vi "Main.vi"(0 "Operation":string(combo), 1 "Delete":bool, 5 "Add":bool, 7 "Load":bool, 9 "Save":bool, 11 "Error In":errorcluster, 12 "Tree":string(tree)) -> (15 "Error Out":errorcluster)   [LabVIEW 2021, in "Calculator.lvlib"]
doc: "This VI acts as a calculator , which has four child classes with the overriding methods and seperate UI VIs for each class which is opened in subpanel when the particular instance is selected. Also the class data is stored in XML file and it can be loaded when required."
uses:
  Calculator.lvlib
  Controls/Queue Operations.ctl
  Classes/NumericOperation/NumericOperation.lvclass
  Controls/Data Cluster.ctl
  Controls/Class Data.ctl
  Controls/User Event Operations.ctl
  <vilib>/Utility/xml.llb/Write to XML File(string).vi
  <vilib>/Utility/xml.llb/Read From XML File(array).vi
panel:
  in  "Help Button":bool
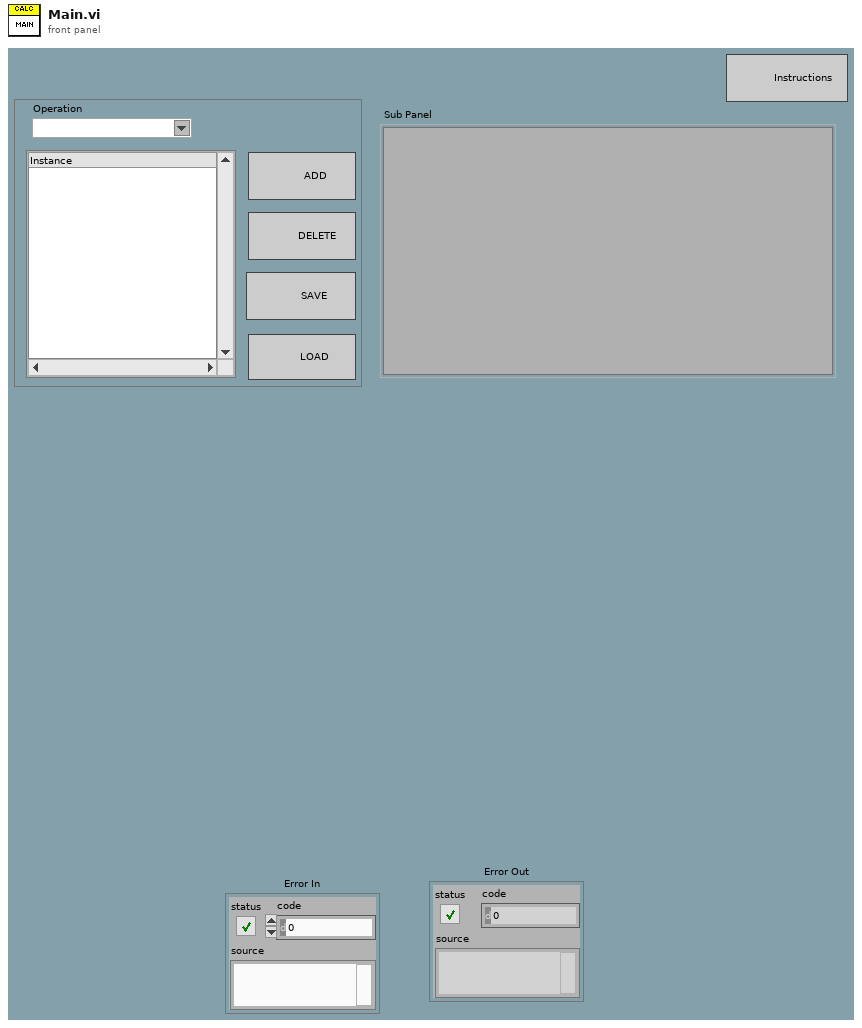
[diagram p1: front panel]
types:
  T1 = typedef "Calculator.lvlib/User Event Operations.ctl" = enum16{"Obtain", "Generate", "Release"}
  T2 = typedef "Calculator.lvlib/Queue Operations.ctl" = enum16{"Create", "Enqueue", "EnqueueN", "Enqueue at top", "Dequeue", "Flush", "Release"}
  T3 = typedef "Calculator.lvlib/Data Cluster.ctl" = cluster{"A":dbl, "B":dbl, "C":dbl, "NumericOperation.lvclass":refnum<class "NumericOperation.lvclass">, "generic class reference":refnum<class "NumericOperation.lvclass">, "Operation":string, "Active Tag":string, "Path":path, "VI Refnum":refnum<vi>, "Class Data":refnum<class "NumericOperation.lvclass">, "DataArray":T4[], "FilePath":path, "Class Name":string, "Data Value Reference Out":refnum<data-value>}
  T4 = typedef "Calculator.lvlib/Class Data.ctl" = cluster{"Class Data":refnum<class "NumericOperation.lvclass">, "String":string}
  T5 = typedef "LVPoint32TypeDef.ctl" = cluster{"Horizontal":i32, "Vertical":i32}
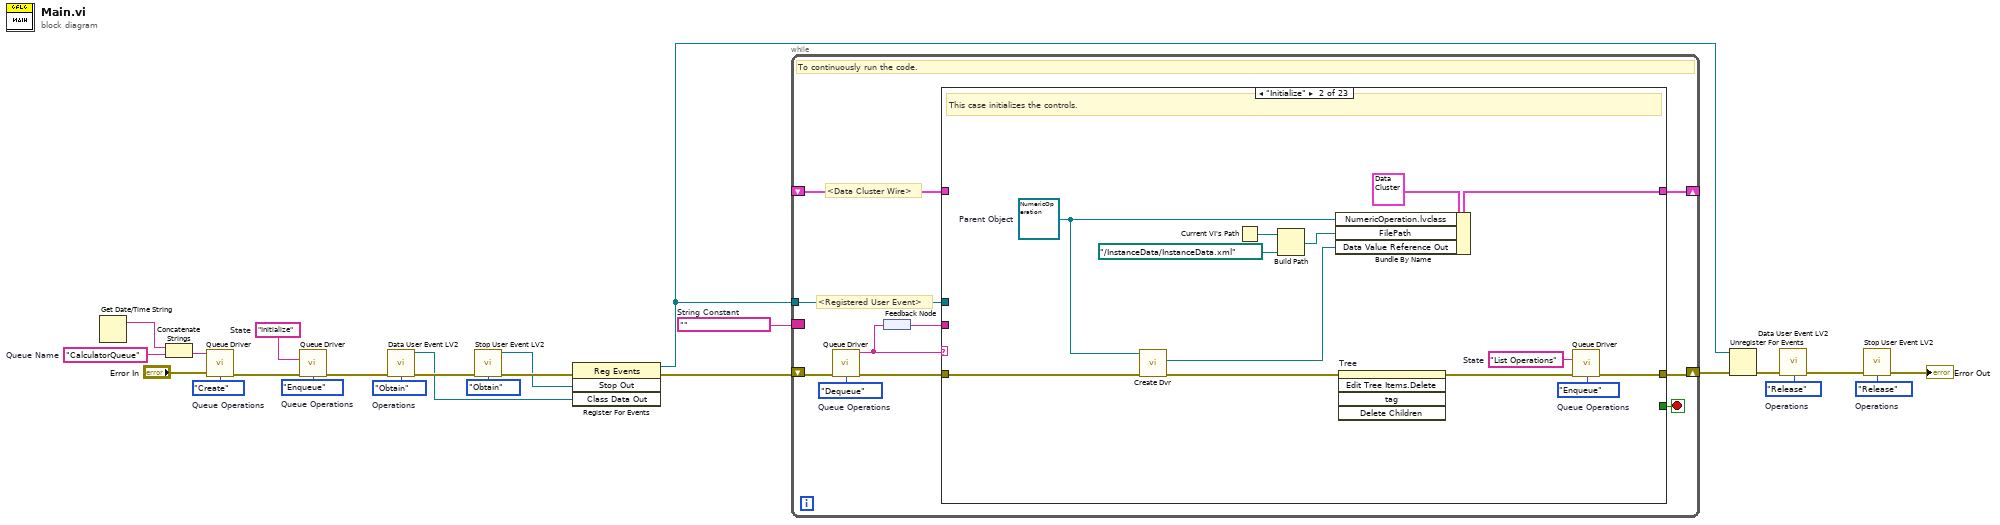
[diagram p0: block diagram]
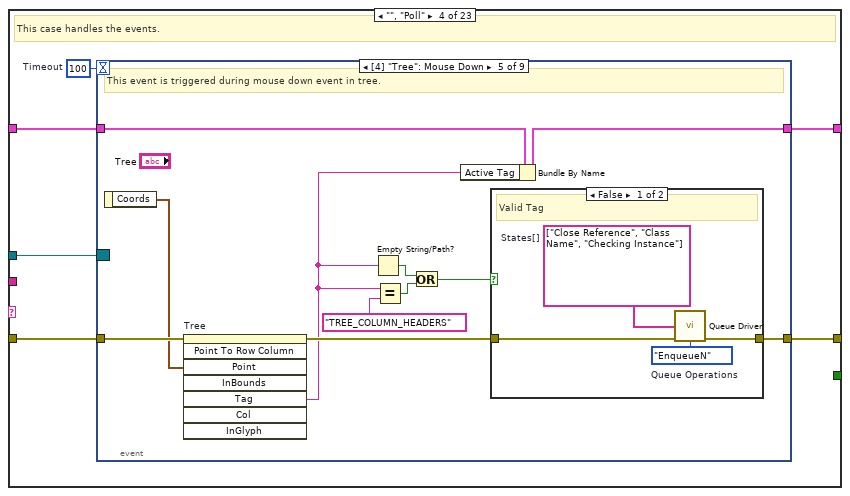
[diagram p4: hidden frame]
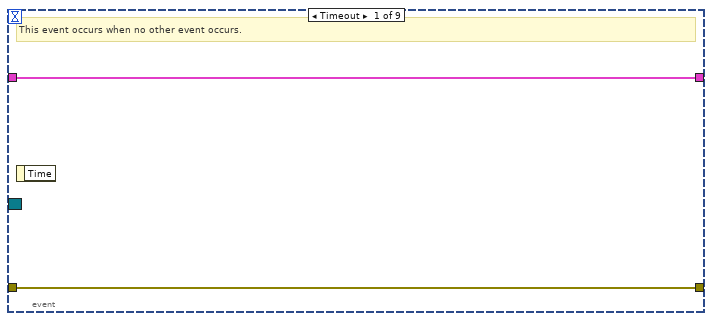
[diagram p5: hidden frame]
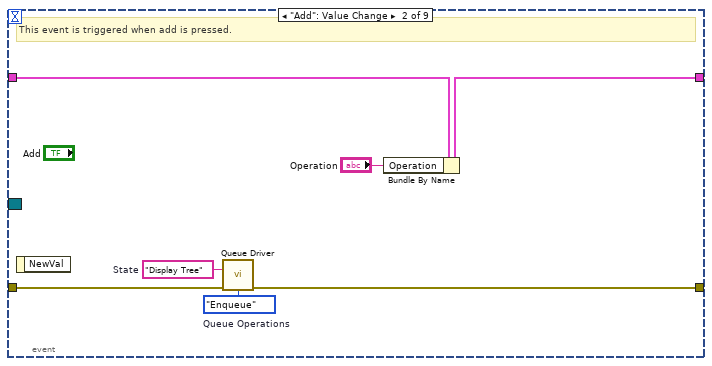
[diagram p6: hidden frame]
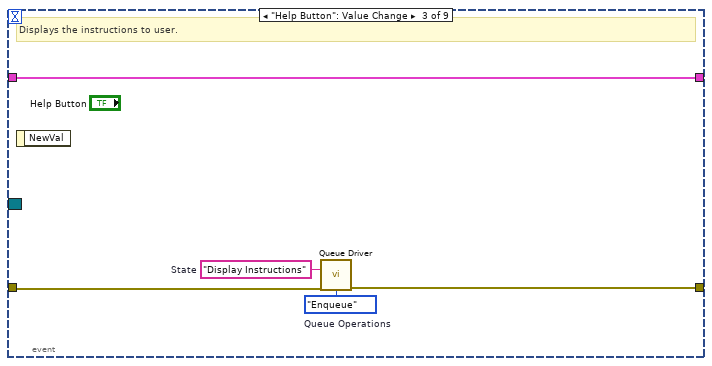
[diagram p7: hidden frame]
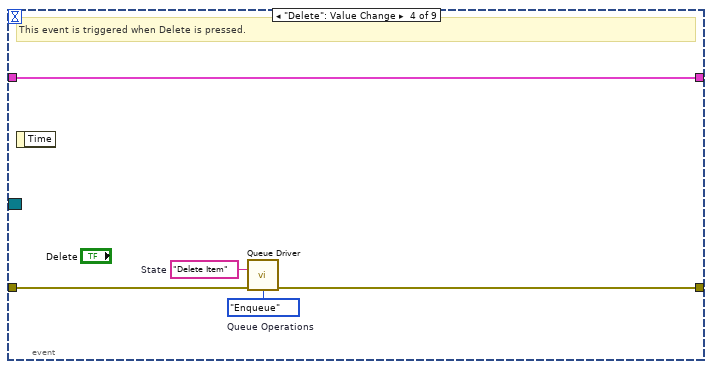
[diagram p8: hidden frame]
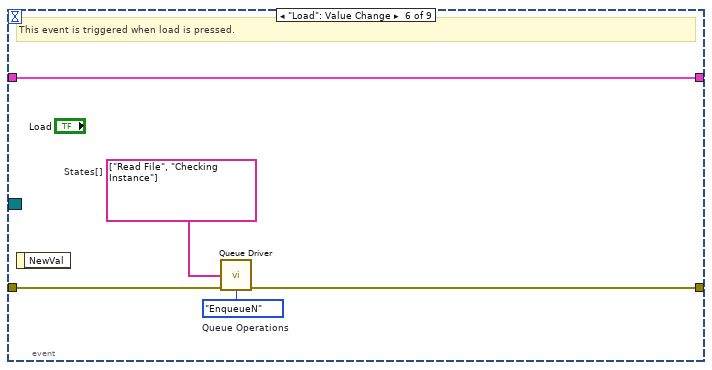
[diagram p10: hidden frame]
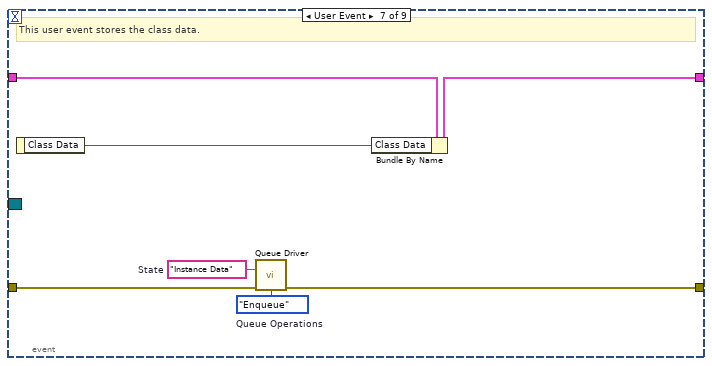
[diagram p11: hidden frame]
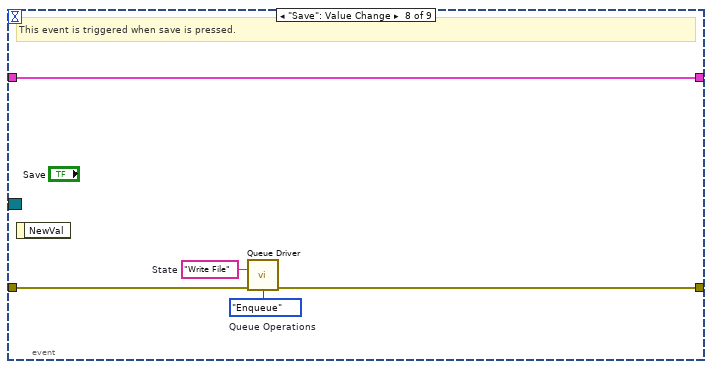
[diagram p12: hidden frame]
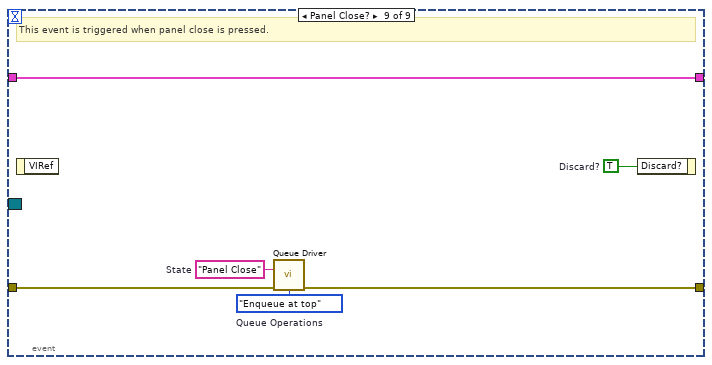
[diagram p13: hidden frame]
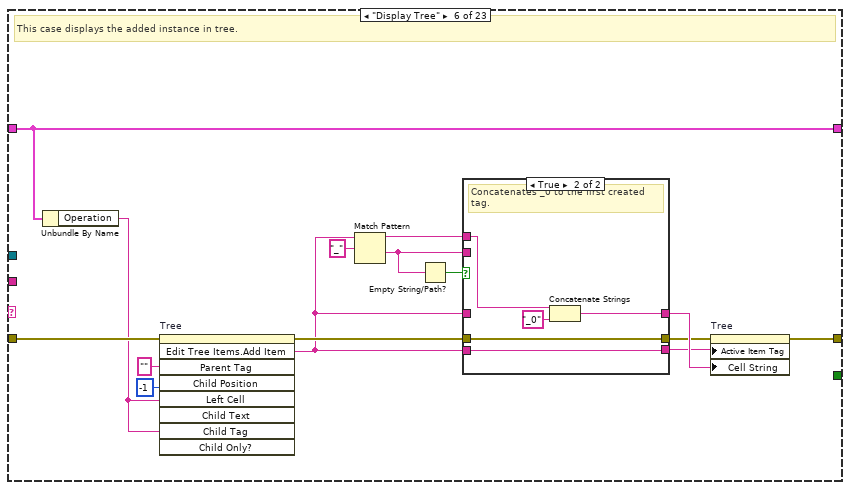
[diagram p15: hidden frame]
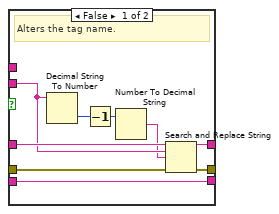
[diagram p16: hidden frame]
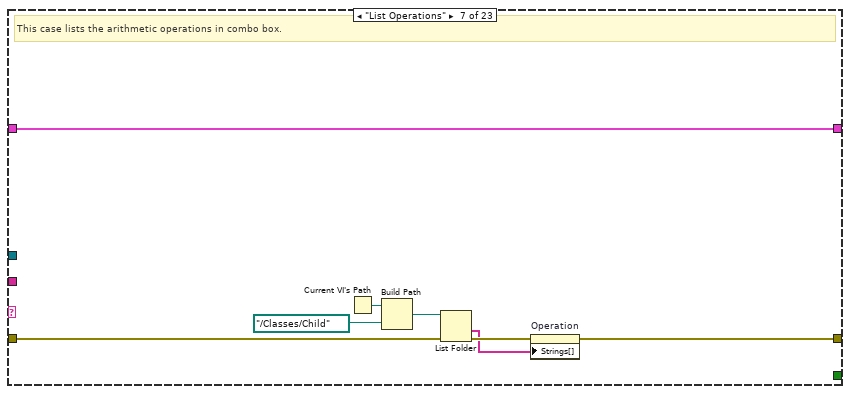
[diagram p17: hidden frame]
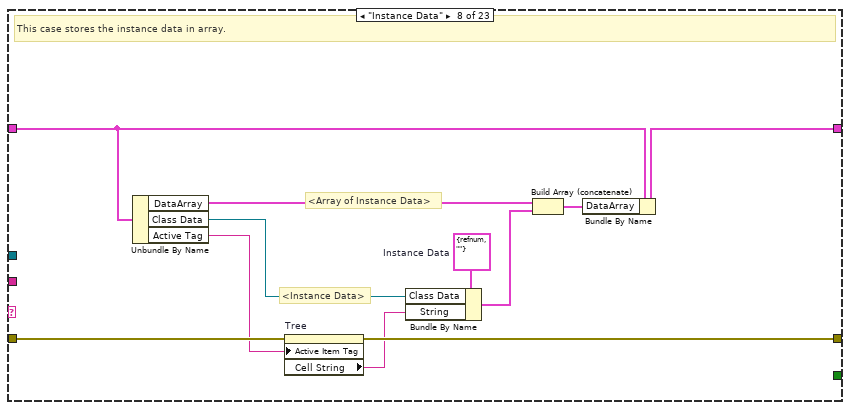
[diagram p18: hidden frame]
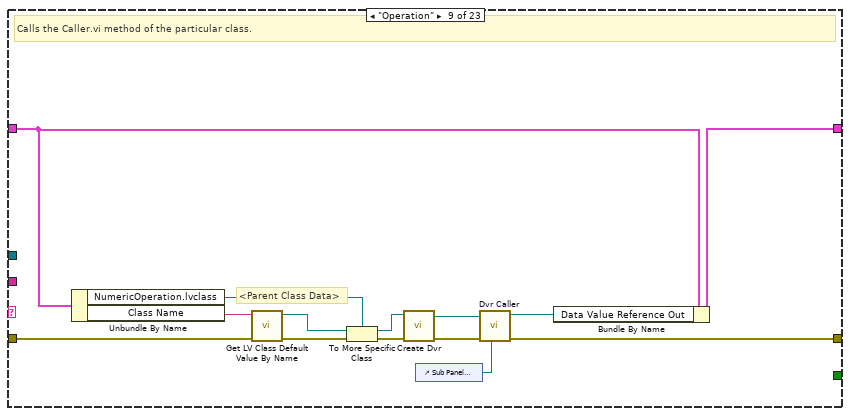
[diagram p19: hidden frame]
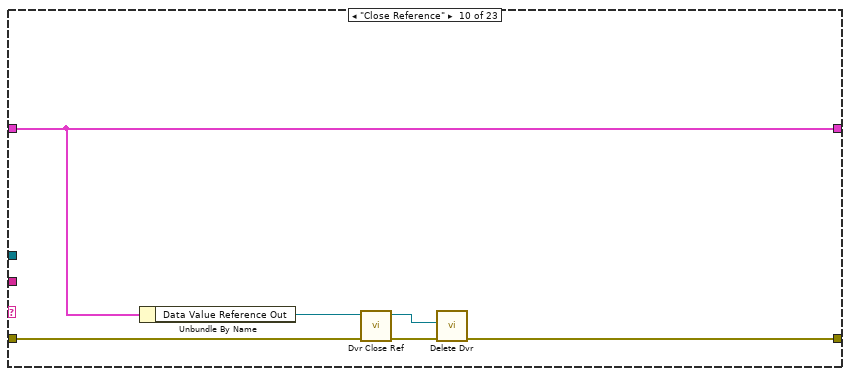
[diagram p20: hidden frame]
diagram:
  w1 = ""  # String Constant
  w2 = User_Event_Operations."Release"  # Operations
  w3 = User_Event_Operations."Release"  # Operations
  w10 = User_Event_Operations."Obtain"  # Operations
  w20 = "Initialize"  # State
  w21 = Queue_Operations."Enqueue"  # Queue Operations
  w18 = "CalculatorQueue"  # Queue Name
  w23 = Queue_Operations."Create"  # Queue Operations
  n1 = Get Date/Time String() -> (date string=w19:string)  [unwired: 3 in, 1 out]
  n2 = Concatenate Strings(w19, w18) -> (w17:string)
  n3 = call "Queue Driver.vi"("Queue Name"=w17, "Error In"="Error In", "Queue Operations"=w23) -> ("Error Out"=w22:errorcluster)  [unwired: 11 in, 1 out]
  n4 = call "Queue Driver.vi"("State"=w20, "Error In"=w22, "Queue Operations"=w21) -> ("Error Out"=w12:errorcluster)  [unwired: 11 in, 1 out]
  n5 = call "Data User Event LV2.vi"("Error In"=w12, "Operations"=w10) -> ("Class Data Out"=w7:refnum<user-event>, "Error Out"=w13:errorcluster)  [unwired: 12 in]
  n6 = call "Stop User Event LV2.vi"("Error In"=w13, "Operations"=User_Event_Operations."Obtain") -> ("Stop Out"=w8:refnum<user-event>, "Error Out"=w11:errorcluster)  [unwired: 12 in]
  n7 = register-events(error in=w11, w8, w7) -> (reference out=w14:refnum<event-registration>, error out=w16:errorcluster)  [unwired: 1 in]
  n8 = while {
    shift-right: [w32] -> _
    shift-left: _ -> [w33]
    shift-right: [w29] -> w15
    shift-left: w16 -> [w30]
    border: w1 -> [_]
    tunnel: w14 -> [w25]
    stop <- w26 stop-if-true
    w34 = Queue_Operations."Dequeue"  # Queue Operations
    # "<Registered User Event>"
    # "<Data Cluster Wire>"
    # "To continuously run the code."
    n9 = call "Queue Driver.vi"("Error In"=w30, "Queue Operations"=w34) -> ("Dequeued Element"=w28:string, "Error Out"=w31:errorcluster)  [unwired: 12 in]
    n10 = feedback-in #1(w28) -> ()
    n11 = feedback #1() -> (w27:string)
    n12 = case shown="\"Initialize\"" w28 {
      tunnel: w33 -> [w36 _ w51 w56 w117 w123 w154 w160 w174 w185 w191 w203 w213 w222 w228 w231 w243 w248 w255 w258 w260 w263 w280]
      tunnel: [w36 w49 w51 w55 w117 w123 w154 w159 w176 w185 w191 w202 w213 w222 w228 w230 w243 w248 w255 w258 w260 w263 w280] -> w32
      tunnel: w31 -> [w35 w40 w50 w54 w116 w132 w150 w165 w175 w184 w188 w200 w214 w221 w225 w236 w242 w247 w254 w257 w259 w262 w279]
      tunnel: [w35 w47 w50 w53 w116 w127 w153 w157 w170 w181 w189 w201 w206 w221 w226 w233 w242 w250 w254 w257 w259 w265 w279] -> w29
      tunnel: w27 -> [_ _ _ _ _ _ _ _ _ _ _ _ _ _ _ _ _ _ _ _ _ w272 _]
      tunnel: [_ _ _ _ _ _ _ _ _ _ _ _ _ _ _ _ _ w249 _ _ _ _ _] -> w26
      tunnel: w25 -> [_ _ _ w52 _ _ _ _ _ _ _ _ _ _ _ _ _ _ _ _ _ _ _]
      frame "/******** Initializing********/" {
        # "Splitter case for initialization."
      }
      frame "Initialize" {
        w45 = "List Operations"  # State
        w46 = Queue_Operations."Enqueue"  # Queue Operations
        w38 = refnum<class "NumericOperation.lvclass"> refnum  # Parent Object
        # "This case initializes the controls."
        n13 = call "Create Dvr.vi"("Error In"=w40, "NumericOperation in"=w38) -> ("Error Out"=w39:errorcluster, "Data Value Reference"=w37:refnum<data-value>)  [unwired: 7 in, 1 out]
        n14 = Current VI's Path() -> (path=w43:path)
        n15 = Build Path(base path=w43, name or relative path=path "../InstanceData/InstanceData.xml") -> (appended path=w48:path)
        n16 = Bundle By Name(cluster=T3 {"A"=0.0, "B"=0.0, "C"=0.0, "NumericOperation.lvclass"=refnum, "generic class reference"=refnum, "Operation"="", "Active Tag"="", "Path"=path "", "VI Refnum"=refnum, "Class Data"=refnum, "DataArray"=[], "FilePath"=path "", "Class Name"="", "Data Value Reference Out"=refnum}, "NumericOperation.lvclass"=w38, "FilePath"=w48, "Data Value Reference Out"=w37) -> (w49:T3)
        n17 = invoke on="Tree" class="Tree (strict)" method="Edit Tree Items.Delete"(error in=w39) -> (error out=w44:errorcluster)  [unwired: 4 in, 4 out]
        n18 = call "Queue Driver.vi"("State"=w45, "Error In"=w44, "Queue Operations"=w46) -> ("Error Out"=w47:errorcluster)  [unwired: 11 in, 1 out]
      }
      frame "/******** Poll ********/" {
        # "Splitter case for poll."
      }
      frame "", "Poll" {
        w57 = 100  # Timeout
        # "This case handles the events."
        n19 = event shown="[4] \"Tree\": Mouse Down" {
          selector: w52 -> [_ _ _ _ _ _ _ _ _]
          dyn-events: _ -> [_ _ _ _ _ _ _ _ _]
          timeout: w57 -> [_ _ _ _ _ _ _ _ _]
          tunnel: w56 -> [w59 w62 w67 w72 w85 w97 w104 w109 w112]
          tunnel: [w59 w61 w67 w72 w84 w97 w102 w109 w112] -> w55
          tunnel: w54 -> [w58 w66 w71 w76 w87 w96 w100 w108 w115]
          tunnel: [w58 w65 w70 w75 w82 w95 w101 w107 w114] -> w53
          event Timeout {
            # "This event occurs when no other event occurs."
            n20 = event-data() -> ()  [unwired: 1 in, 1 out]
          }
          event "Add": Value Change {
            w63 = "Display Tree"  # State
            w64 = Queue_Operations."Enqueue"  # Queue Operations
            # "This event is triggered when add is pressed."
            n21 = event-data() -> ()  [unwired: 1 in, 1 out]
            n22 = call "Queue Driver.vi"("State"=w63, "Error In"=w66, "Queue Operations"=w64) -> ("Error Out"=w65:errorcluster)  [unwired: 11 in, 1 out]
            n23 = Bundle By Name(cluster=w62, "Operation"="Operation") -> (w61:T3)
          }
          event "Help Button": Value Change {
            w68 = "Display Instructions"  # State
            w69 = Queue_Operations."Enqueue"  # Queue Operations
            # "Displays the instructions to user."
            n24 = event-data() -> ()  [unwired: 1 in, 1 out]
            n25 = call "Queue Driver.vi"("State"=w68, "Error In"=w71, "Queue Operations"=w69) -> ("Error Out"=w70:errorcluster)  [unwired: 11 in, 1 out]
          }
          event "Delete": Value Change {
            w73 = "Delete Item"  # State
            w74 = Queue_Operations."Enqueue"  # Queue Operations
            # "This event is triggered when Delete is pressed."
            n26 = event-data() -> ()  [unwired: 1 in, 1 out]
            n27 = call "Queue Driver.vi"("State"=w73, "Error In"=w76, "Queue Operations"=w74) -> ("Error Out"=w75:errorcluster)  [unwired: 11 in, 1 out]
          }
          event "Tree": Mouse Down {
            # "This event is triggered during mouse down event in tree."
            n28 = event-data() -> ("Coords"=w86:T5)  [unwired: 1 in]
            n29 = invoke on="Tree" class="Tree (strict)" method="Point To Row Column"(error in=w87, "Point"=w86) -> (error out=w83:errorcluster, "Tag"=w81:string)  [unwired: 6 in, 6 out]
            n30 = Empty String/Path?(string/path=w81) -> (empty?=w78:bool)
            n31 = Equal?(x=w81, y="TREE_COLUMN_HEADERS") -> (x = y?=w79:bool)
            n32 = Or(x=w78, y=w79) -> (x .or. y?=w77:bool)
            n33 = Bundle By Name(cluster=w85, "Active Tag"=w81) -> (w84:T3)
            n34 = case shown="False" w77 {
              tunnel: w83 -> [w91 w92]
              tunnel: [w90 w92] -> w82
              frame False {
                w88 = string[] ["Close Reference", "Class Name", "Checking Instance"]  # States[]
                w89 = Queue_Operations."EnqueueN"  # Queue Operations
                # "Valid Tag"
                n35 = call "Queue Driver.vi"("States[]"=w88, "Error In"=w91, "Queue Operations"=w89) -> ("Error Out"=w90:errorcluster)  [unwired: 11 in, 1 out]
              }
              frame True {
                # "Invalid Tag"
              }
            }
          }
          event "Load": Value Change {
            w93 = string[] ["Read File", "Checking Instance"]  # States[]
            w94 = Queue_Operations."EnqueueN"  # Queue Operations
            # "This event is triggered when load is pressed."
            n36 = event-data() -> ()  [unwired: 1 in, 1 out]
            n37 = call "Queue Driver.vi"("States[]"=w93, "Error In"=w96, "Queue Operations"=w94) -> ("Error Out"=w95:errorcluster)  [unwired: 11 in, 1 out]
          }
          event User Event {
            w98 = "Instance Data"  # State
            w99 = Queue_Operations."Enqueue"  # Queue Operations
            # "This user event stores the class data."
            n38 = event-data() -> ("Class Data"=w103:refnum<class "NumericOperation.lvclass">)  [unwired: 1 in]
            n39 = call "Queue Driver.vi"("State"=w98, "Error In"=w100, "Queue Operations"=w99) -> ("Error Out"=w101:errorcluster)  [unwired: 11 in, 1 out]
            n40 = Bundle By Name(cluster=w104, "Class Data"=w103) -> (w102:T3)
          }
          event "Save": Value Change {
            w105 = "Write File"  # State
            w106 = Queue_Operations."Enqueue"  # Queue Operations
            # "This event is triggered when save is pressed."
            n41 = event-data() -> ()  [unwired: 1 in, 1 out]
            n42 = call "Queue Driver.vi"("State"=w105, "Error In"=w108, "Queue Operations"=w106) -> ("Error Out"=w107:errorcluster)  [unwired: 11 in, 1 out]
          }
          event Panel Close? {
            w111 = Queue_Operations."Enqueue at top"  # Queue Operations
            w113 = "Panel Close"  # State
            w110 = TRUE  # Discard?
            # "This event is triggered when panel close is pressed."
            n43 = event-data() -> ()  [unwired: 1 in, 1 out]
            n44 = call "Queue Driver.vi"("State"=w113, "Error In"=w115, "Queue Operations"=w111) -> ("Error Out"=w114:errorcluster)  [unwired: 11 in, 1 out]
            n45 = event-data("Discard?"=w110) -> ()  [unwired: 1 in, 1 out]
          }
        }
      }
      frame "/******** Functionalities ********/" {
        # "Splitter case for functionalities."
      }
      frame "Display Tree" {
        # "This case displays the added instance in tree."
        n46 = Unbundle By Name(w123) -> ("Operation"=w122:string)
        n47 = invoke on="Tree" class="Tree (strict)" method="Edit Tree Items.Add Item"(error in=w132, "Parent Tag"="", "Child Position"=-1, "Left Cell"=w122, "Child Tag"=w122) -> (error out=w121:errorcluster, "Edit Tree Items:Add Item"=w119:string)  [unwired: 4 in, 7 out]
        n48 = Match Pattern(string=w119, regular expression="_") -> (before substring=w128:string, after substring=w124:string)  [unwired: 1 in, 2 out]
        n49 = Empty String/Path?(string/path=w124) -> (empty?=w125:bool)
        n50 = case shown="True" w125 {
          tunnel: [w138 w145] -> w126
          tunnel: w128 -> [_ w144]
          tunnel: w124 -> [w139 _]
          tunnel: w119 -> [w140 _]
          tunnel: w121 -> [w135 w143]
          tunnel: [w134 w143] -> w120
          tunnel: [w133 w142] -> w118
          tunnel: w119 -> [w133 w142]
          frame False {
            # "Alters the tag name."
            n51 = Decimal String To Number(string=w139) -> (number=w137:i32)  [unwired: 2 in, 1 out]
            n52 = Decrement(x=w137) -> (x-1=w141:i32)
            n53 = Number To Decimal String(number=w141) -> (decimal integer string=w136:string)  [unwired: 1 in]
            n54 = Search and Replace String(input string=w140, search string=w139, replace string=w136, error in=w135) -> (result string=w138:string, error out=w134:errorcluster)  [unwired: 4 in, 2 out]
          }
          frame True {
            # "Concatenates _0 to the first created tag."
            n55 = Concatenate Strings(w144, "_0" ("string")) -> (w145:string)
          }
        }
        n56 = property on="Tree" class="Tree (strict)"(error in=w120, "Active Item Tag"=w118, "Cell String"=w126) -> (error out=w127:errorcluster)  [unwired: 1 in, 1 out]
      }
      frame "List Operations" {
        # "This case lists the arithmetic operations in combo box."
        n57 = Current VI's Path() -> (path=w152:path)
        n58 = Build Path(base path=w152, name or relative path=path "../Classes/Child") -> (appended path=w148:path)
        n59 = List Folder(path=w148, error in=w150) -> (folder names=w147:string[], error out=w149:errorcluster)  [unwired: 2 in, 2 out]
        n60 = property on="Operation" class="CmbBox"(error in=w149, "Strings[]"=w147) -> (error out=w153:errorcluster)  [unwired: 1 in, 1 out]
      }
      frame "Instance Data" {
        w164 = T4 {"Class Data"=refnum, "String"=""}  # Instance Data
        # "<Instance Data>"
        # "<Array of Instance Data>"
        # "This case stores the instance data in array."
        n61 = Unbundle By Name(w160) -> ("DataArray"=w162:T4[], "Class Data"=w163:refnum<class "NumericOperation.lvclass">, "Active Tag"=w156:string)
        n62 = property on="Tree" class="Tree (strict)"(error in=w165, "Active Item Tag"=w156) -> (error out=w157:errorcluster, "Cell String"=w155:string)  [unwired: 1 in, 1 out]
        n63 = Bundle By Name(cluster=w164, "Class Data"=w163, "String"=w155) -> (w161:T4)
        n64 = Build Array (concatenate)(w162, w161) -> (w158:T4[])
        n65 = Bundle By Name(cluster=w160, "DataArray"=w158) -> (w159:T3)
      }
      frame "Operation" {
        # "<Parent Class Data>"
        # "Calls the Caller.vi method of the particular class."
        n66 = Unbundle By Name(w174) -> ("NumericOperation.lvclass"=w173:refnum<class "NumericOperation.lvclass">, "Class Name"=w177:string)
        n67 = call <vilib>:"Get LV Class Default Value By Name.vi"("error in (no error)"=w175, "class name"=w177) -> ("error out"=w178:errorcluster, "object"=w179:refnum<class>)  [unwired: 8 in]
        n68 = To More Specific Class(target class=w173, reference=w179, error in=w178) -> (specific class reference=w169:refnum<class "NumericOperation.lvclass">, error out=w171:errorcluster)
        n69 = call "Create Dvr.vi"("Error In"=w171, "NumericOperation in"=w169) -> ("Error Out"=w172:errorcluster, "Data Value Reference"=w168:refnum<data-value>)  [unwired: 7 in, 1 out]
        n70 = control-ref of="Sub Panel Reference"() -> (w167:refnum<vi>)
        n71 = call "Dvr Caller.vi"("Sub Panel"=w167, "Error In"=w172, "Data Value Reference In"=w168) -> ("Error Out"=w170:errorcluster, "Data Value Reference Out"=w166:refnum<data-value>)  [unwired: 7 in]
        n72 = Bundle By Name(cluster=w174, "Data Value Reference Out"=w166) -> (w176:T3)
      }
      frame "Close Reference" {
        n73 = Unbundle By Name(w185) -> ("Data Value Reference Out"=w183:refnum<data-value>)
        n74 = call "Dvr Close Ref.vi"("Error In"=w184, "Data Value Reference In"=w183) -> ("Error Out"=w182:errorcluster, "Data Value Reference Out"=w180:refnum<data-value>)  [unwired: 8 in]
        n75 = call "Delete Dvr.vi"("Error In"=w182, "Data Value Reference"=w180) -> ("Error Out"=w181:errorcluster)  [unwired: 9 in]
      }
      frame "Delete Item" {
        # "Deletes the item from tree."
        n76 = property on="Tree" class="Tree (strict)"(error in=w188) -> (error out=w187:errorcluster, "Value"=w186:string)  [unwired: 1 in, 1 out]
        n77 = invoke on="Tree" class="Tree (strict)" method="Edit Tree Items.Delete"(error in=w187, "tag"=w186) -> (error out=w190:errorcluster)  [unwired: 3 in, 4 out]
        n78 = invoke on="Sub Panel" class="SubPnl" method="Remove VI"(error in=w190) -> (error out=w189:errorcluster)  [unwired: 2 in, 2 out]
      }
      frame "Class Name" {
        w194 = Queue_Operations."Enqueue at top"  # Queue Operations
        # "Gives the class name of the active instance."
        n79 = Unbundle By Name(w203) -> ("Active Tag"=w199:string)
        n80 = Match Pattern(string=w199, regular expression="_") -> (before substring=w197:string)  [unwired: 1 in, 3 out]
        n81 = Concatenate Strings("Calculator.lvlib:" ("string"), w197, ".lvclass" ("string")) -> (w195:string)
        n82 = Bundle By Name(cluster=w203, "Class Name"=w195) -> (w202:T3)
        n83 = call "Queue Driver.vi"("State"="Operation", "Error In"=w200, "Queue Operations"=w194) -> ("Error Out"=w201:errorcluster)  [unwired: 11 in, 1 out]
      }
      frame "Checking Instance" {
        w204 = User_Event_Operations."Generate"  # Operations
        # "Gives the recent data of active instance that is stored in array."
        n84 = Unbundle By Name(w213) -> ("DataArray"=w209:T4[], "Active Tag"=w211:string)
        n85 = property on="Tree" class="Tree (strict)"(error in=w214, "Active Item Tag"=w211) -> (error out=w212:errorcluster, "Cell String"=w210:string)  [unwired: 1 in, 1 out]
        n86 = Reverse 1D Array(array=w209) -> (reversed array=w208:T4[])
        n87 = for {
          tunnel: w210 -> [w219]
          tunnel: w208 -> [w217] mode=indexing
          tunnel: [w216] -> w205 if=w215
          shift-right: [w218] -> w207
          shift-left: w212 -> [w218]
          stop <- w215 stop-if-true
          # "Search for the recent instance from array"
          n88 = Unbundle By Name(w217) -> ("Class Data"=w216:refnum<class "NumericOperation.lvclass">, "String"=w220:string)
          n89 = Equal?(x=w220, y=w219) -> (x = y?=w215:bool)
        }
        n90 = call "Data User Event LV2.vi"("Class Data"=w205, "Error In"=w207, "Operations"=w204) -> ("Error Out"=w206:errorcluster)  [unwired: 11 in, 1 out]
      }
      frame "/******** File Operations ********/" {
        # "Splitter case for File Operations."
      }
      frame "Write File" {
        # "Flattens the class data and write it to the XML file."
        n91 = Unbundle By Name(w228) -> ("FilePath"=w227:path, "DataArray"=w224:T4[])
        n92 = Flatten To XML(6:w224) -> (2:w223:string)
        n93 = call-poly <vilib>:"Write to XML File.vi"("error in (no error)"=w225, "XML Input"=w223, "XML File Path"=w227) -> ("error out"=w226:errorcluster)  [unwired: 6 in, 2 out]
      }
      frame "Read File" {
        # "Reads the stored data from XML file and unflattens the data to store in array."
        n94 = Unbundle By Name(w231) -> ("FilePath"=w235:path)
        n95 = call-poly <vilib>:"Read From XML File.vi"("error in (no error)"=w236, "XML File Path"=w235) -> ("error out"=w234:errorcluster, "XML Elements"=w232:string[])  [unwired: 7 in, 1 out]
        n96 = for {
          shift-right: [w240] -> w233
          shift-left: w234 -> [w241]
          tunnel: w232 -> [w238] mode=indexing
          tunnel: [w239] -> w229 mode=concatenating
          w237 = T4[] []  # Array of Instance Data
          # "Unflattens the data."
          n97 = Unflatten From XML(xml string=w238, type=w237, error in (no error)=w241) -> (value=w239:T4[], error out=w240:errorcluster)
        }
        n98 = Bundle By Name(cluster=w231, "DataArray"=w229) -> (w230:T3)
      }
      frame "/******** Panel Close ********/" {
        # "Splitter case for Panel Close."
      }
      frame "Panel Close" {
        w244 = TRUE  # Stop?
        w245 = User_Event_Operations."Generate"  # Operations
        w249 = TRUE  # Exit?
        w252 = Queue_Operations."Release"  # Queue Operations
        w253 = Queue_Operations."Flush"  # Queue Operations
        # "Stops the running VI ."
        n99 = call "Stop User Event LV2.vi"("Stop"=w244, "Error In"=w247, "Operations"=w245) -> ("Error Out"=w246:errorcluster)  [unwired: 11 in, 1 out]
        n100 = call "Queue Driver.vi"("Error In"=w246, "Queue Operations"=w253) -> ("Error Out"=w251:errorcluster)  [unwired: 12 in, 1 out]
        n101 = call "Queue Driver.vi"("Error In"=w251, "Queue Operations"=w252) -> ("Error Out"=w250:errorcluster)  [unwired: 12 in, 1 out]
      }
      frame "/******* Display Instruction ********/" {
        # "Splitter case for instruction display."
      }
      frame "Display Instructions" {
        n102 = One Button Dialog(message="INSTRUCTIONS :\n\n1. Select the Operation from the combo box.\n2. Press ADD to add the instance in tree.\n3. Click the added instance in tree and it opens in the subpanel.\n4. Enter the inputs and press calculate.\n5. Press SAVE to save the data in XML file after calculating for a particular instance.\n6. Press LOAD to load the saved data of instances from XML file.\n7. Select the instance to delete and press DELETE to delete that particular instance.\n") -> ()  [unwired: 1 in, 1 out]
      }
      frame "/******** Error Handling ********/" {
        # "Splitter case for Error Handling"
      }
      frame "Error" {
        # "This case handles the error."
        n103 = Unbundle By Name(w262) -> ("code"=w271:i32, "source"=w270:string)
        n104 = call <vilib>:"Clear Errors.vi"("error in (no error)"=w262) -> ("error out"=w261:errorcluster)  [unwired: 5 in, 1 out]
        n105 = Format Into String(format string="Error occurred in state \"%s\"!!\nError Code: %d\nError Source: %s\n\nDo you wish to continue?", error in=w261, w272, w271, w270) -> (resulting string=w267:string, error out=w266:errorcluster)  [unwired: 1 in]
        n106 = Two Button Dialog(message=w267, 1:"Exit" ("F button name (\"Cancel\")"), 2:"Continue" ("T button name (\"OK\")")) -> (T button?=w264:bool)
        n107 = case "Continue?" shown="False" w264 {
          tunnel: w266 -> [w277 w278]
          tunnel: [w276 w278] -> w265
          frame False {
            w275 = "Panel Close"  # State
            # "This case occurs when exit is pressed."
            n108 = call "Queue Driver.vi"("State"=w275, "Error In"=w277, "Queue Operations"=Queue_Operations."Enqueue at top") -> ("Error Out"=w276:errorcluster)  [unwired: 11 in, 1 out]
          }
          frame True {
            # "This case occurs when continue is pressed."
          }
        }
      }
      frame Default {
        # "Developer error."
      }
    }
  }
  n109 = Unregister For Events(event registration refnum=w14, error in=w15) -> (error out=w5:errorcluster)
  n110 = call "Data User Event LV2.vi"("Error In"=w5, "Operations"=w3) -> ("Error Out"=w6:errorcluster)  [unwired: 12 in, 1 out]
  n111 = call "Stop User Event LV2.vi"("Error In"=w6, "Operations"=w2) -> ("Error Out"=→"Error Out":errorcluster)  [unwired: 12 in, 1 out]
